vi "Autocycle v0.1.vi"(6 "start time":timestamp, 7 "Message Queue":refnum<queue>, 8 "error in":errorcluster, 9 "Run Time in":dbl, 10 "Auto Para":T1={"Agitator Delays"=[], "TF Delays"=[], "Insertion Delays"=[], "Cutting Delays"=[], "PF Delays"=[], "Measur. Delays"=[1000.0], "Reject Delays"=[1000], "BF Delays"=[1000]}, 11 "Counts in":cluster{"OutputCount":u32, "RejectCount":u32}) -> (0 "error out":errorcluster, 1 "Run Time out":dbl, 3 "Counts out":cluster{"OutputCount":u32, "RejectCount":u32})   [LabVIEW 2017]
uses:
  Controls/Auto Delays.ctl
  support/Message Queue/Message Cluster.ctl
  Controls/Auto Times.ctl
  Global Variables/RT GV.vi
  Global Variables/FPGA GV.vi
  <vilib>/Utility/error.llb/Error Cluster From Error Code.vi
  <vilib>/rvi/errors/niLvFpgaAdjustHostInterfaceError.vi
  support/Message Queue/Enqueue Message (Single).vi
  <vilib>/rvi/interface/nirviReadWriteControl/nirviReadWriteControl.xnode
  Controls/FPGA Ref.ctl
  NiFpgaLv.dll
  <vilib>/rvi/interface/Simulation/niFpgaSimulationCallBeginRW.vi
  support/Message Queue/Message Queue.lvlib
panel:
  in  "Max Successive":u32
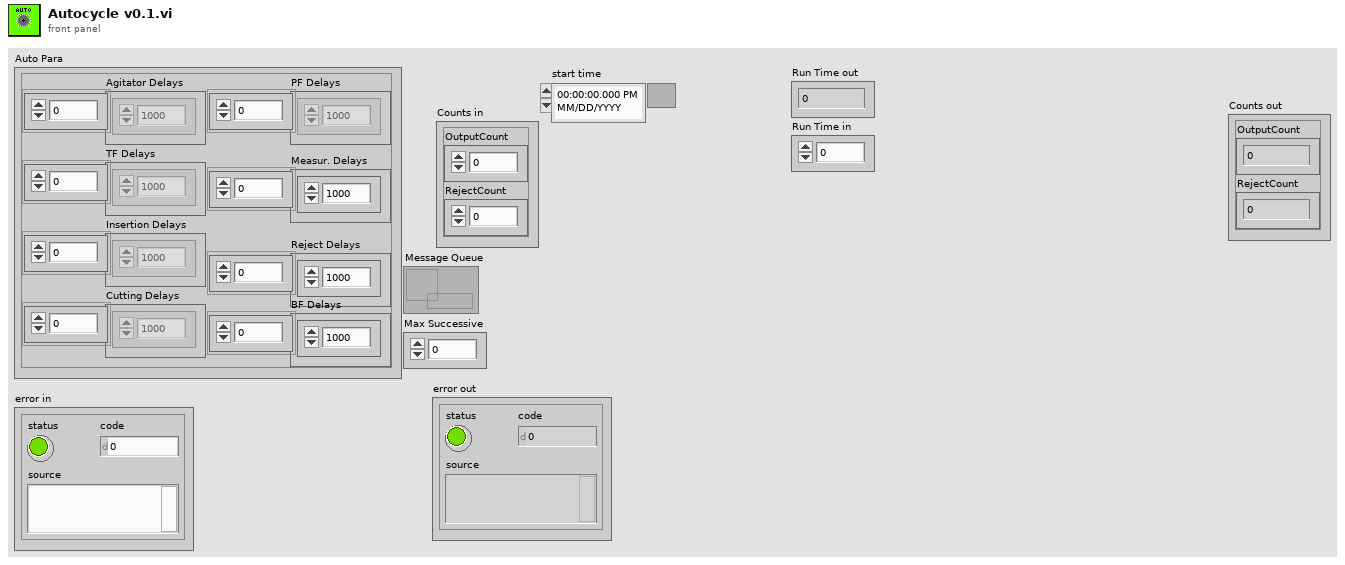
[diagram p1: front panel]
types:
  T1 = typedef "Auto Delays.ctl" = cluster{"Agitator Delays":u32[], "TF Delays":u32[], "Insertion Delays":u32[], "Cutting Delays":u32[], "PF Delays":u32[], "Measur. Delays":dbl[], "Reject Delays":u32[], "BF Delays":u32[]}
  T2 = cluster{"Tube Present":bool[], "Output Count":u32}
  T3 = typedef "FPGA Ref.ctl" = refnum<k20>
  T4 = cluster{"TL_Red":bool, "TL_Orange":bool, "TL_Green":bool, "TL_Buzzer":bool, "SOL_Index_Rotary_CW":bool, "SOL_Index_CNVR_Rotary_CCW":bool, "SOL_Index_CNVR_Stopper_Rear":bool, "SOL_Index_CNVR_Output _Separator _Rear":bool, "Bowl Feeder_ ON1":bool, "Pump_CNVR_Motor _ON":bool, "SOL_PC_Gating_CYL_Rear":bool, "SOL_Tube_Feed_Agitatator":bool, "SOL_Tube_Feed_Gating_CYL":bool, "SOL_Insertion _CYL":bool, "SOL_Insertion_Clamp_CYL":bool, "SOL_Cutting_CYL":bool, "SOL_Cutting_Clamp_CYL":bool, "SOL_Insertion_Air_Nozzle":bool, "SOL_Measurement_CYL":bool, "DO1.19":bool, "SOL_Rejection CYL_1":bool, "SOL_Rejection CYL_2":bool, "SOL_Rejection CYL_3":bool, "SOL_Rejection CYL_4":bool, "Bowl Feeder_ON2":bool, "SOL_BF_BlowerON":bool, "SOL_BF1_Track1":bool, "SOL_BF1_Track2":bool, "SOL_BF2_Track1":bool, "SOL_BF2_Track2":bool, "DO1.30":bool, "DO1.31":bool}
  T5 = cluster{"Indexes":i32, "seconds since 1Jan1904":timestamp}
  T6 = typedef "Auto Times.ctl" = cluster{"Index Time":u32, "TF Time":u32, "Insertion Time":u32, "Cutting Time":u32, "PF Time":u32, "Meas. Time":u32, "Reject Time":u32}
  T7 = cluster{"Reject 1":bool, "Reject 2":bool, "Reject 3":bool, "Reject 4":bool}
  T8 = cluster{"Tube Present":bool[], "Parts Count":u32}
  T9 = cluster{"seconds since 1Jan1904":timestamp, "Auto Times":T6, "start time":timestamp}
  T10 = cluster{"Reject Pallets":cluster{"Reject 1":bool, "Reject 2":bool, "Reject 3":bool, "Reject 4":bool}, "Measurements":cluster{"1":dbl, "2":dbl, "3":dbl, "4":dbl}}
  T11 = typedef "Auto Stats.ctl" = cluster{"Time":timestamp, "OEE":cluster{"AVL":dbl, "PRF":dbl, "QUA":dbl, "OEE":dbl}, "Auto Times":T6, "Counts out":cluster{"OutputCount":u32, "RejectCount":u32}, "Measurements":cluster{"1":dbl, "2":dbl, "3":dbl, "4":dbl}, "Outputs":cluster{"OutputCount":u32, "Numeric Control":u32}}
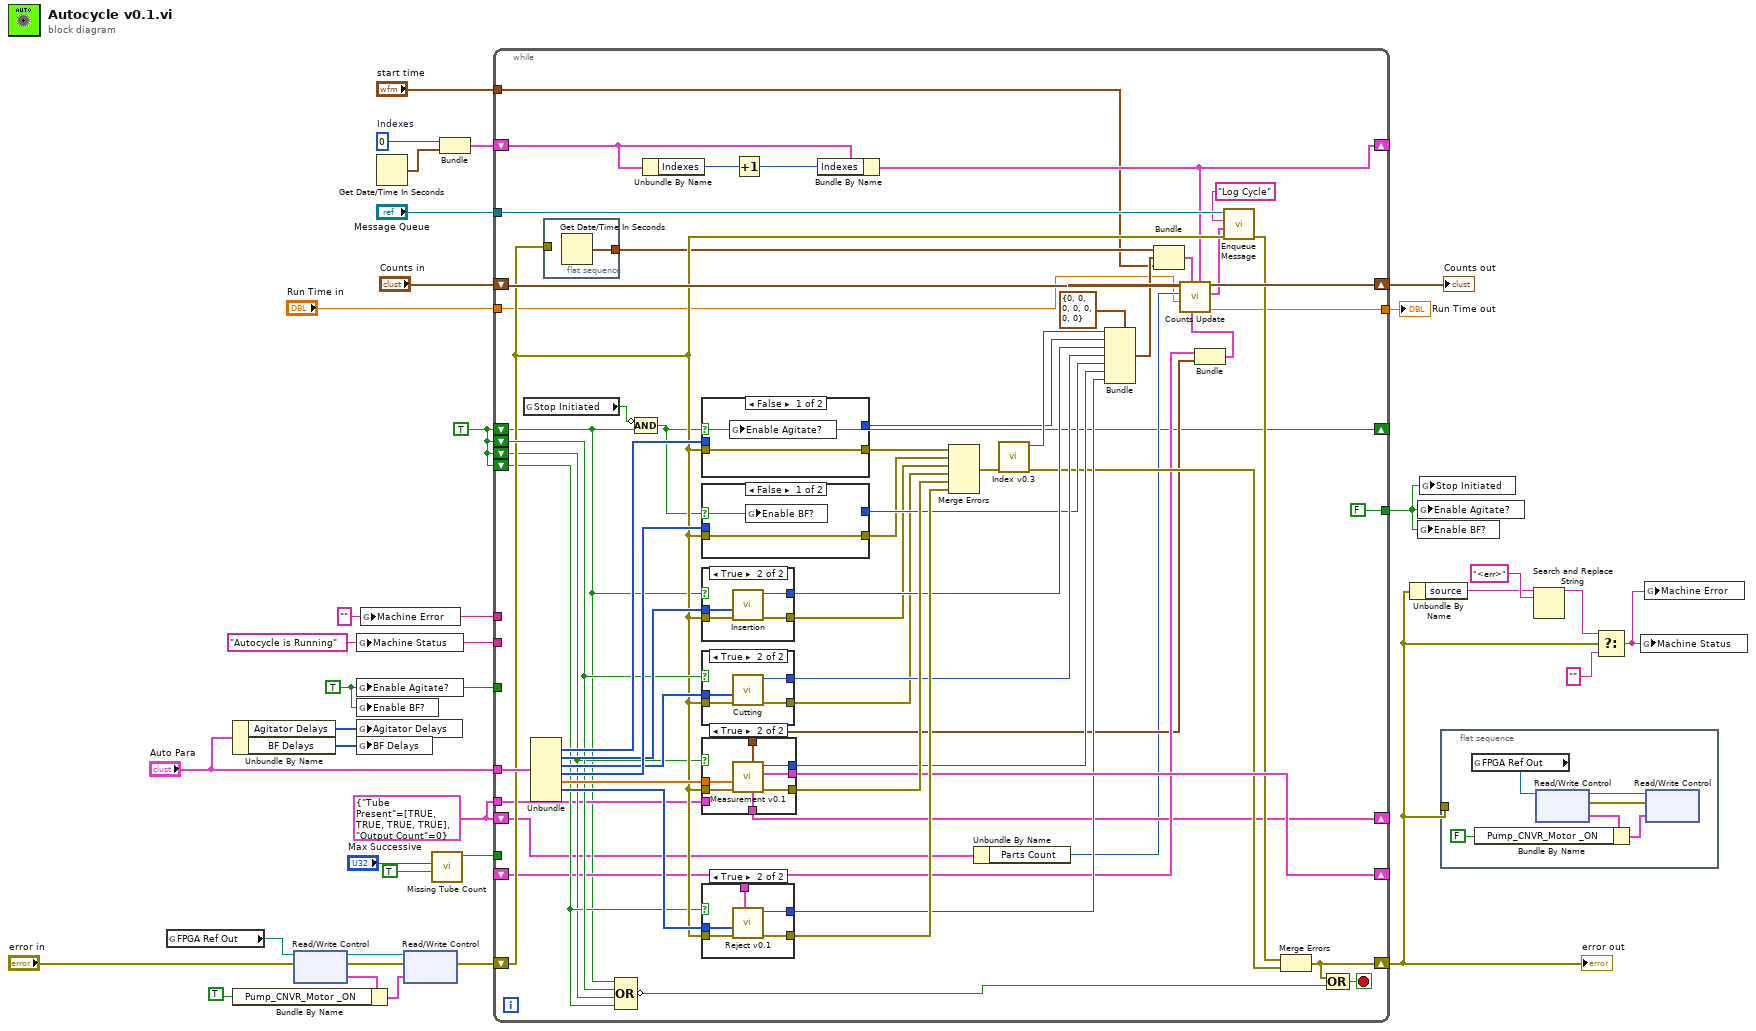
[diagram p0: block diagram]
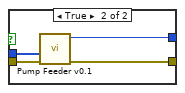
[diagram p2: hidden frame]
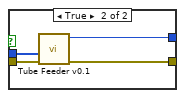
[diagram p5: hidden frame]
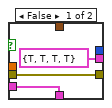
[diagram p7: hidden frame]
diagram:
  w7 = T2 {"Tube Present"=[TRUE, TRUE, TRUE, TRUE], "Output Count"=0} ("Part Count")
  w8 = "" ("Machine Error")
  w13 = 0  # Indexes
  w19 = "Autocycle is Running" ("Machine Status")
  w30 = TRUE ("Enable Agitate?")
  w20 = TRUE
  n1 = global read "FPGA GV.vi" "FPGA Ref Out"() -> (w29:T3)
  n2 = Unbundle By Name("Auto Para") -> ("Agitator Delays"=w32:u32[], "BF Delays"=w31:u32[])
  n3 = xnode "Read/Write Control"("FPGA VI Reference In"=w29, "error in"="error in") -> ("FPGA VI Reference Out"=w24:T3, "error out"=w25:errorcluster, "DO 1"=w28:T4)
  n4 = Bundle By Name(cluster=w28, "Pump_CNVR_Motor _ON"=TRUE) -> (w27:T4)
  n5 = global write "RT GV.vi" "Machine Status"(w19) -> ()
  n6 = global write "RT GV.vi" "Enable Agitate?"(w30) -> ()
  n7 = global write "RT GV.vi" "Enable BF?"(w30) -> ()
  n8 = global write "RT GV.vi" "Agitator Delays"(w32) -> ()
  n9 = global write "RT GV.vi" "BF Delays"(w31) -> ()
  n10 = global write "RT GV.vi" "Machine Error"(w8) -> ()
  n11 = Get Date/Time In Seconds() -> (seconds since 1Jan1904=w12:timestamp)
  n12 = xnode "Read/Write Control"("FPGA VI Reference In"=w24, "error in"=w25, "DO 1"=w27) -> ("error out"=w22:errorcluster)  [unwired: 1 out]
  n13 = call "Missing Tube Count.vi"("ResetMT?"=TRUE, "Max Successive"="Max Successive") -> ("Boolean"=w1:bool)  [unwired: 9 in]
  n14 = Bundle("Indexes"=w13, "seconds since 1Jan1904"=w12) -> (w11:T5)  [unwired: 1 in]
  n15 = while {
    tunnel: "Auto Para" -> [w89]
    shift-right: [w60] -> w17
    shift-left: w22 -> [w62]
    shift-right: [w83] -> _
    shift-left: _ -> [w54]
    shift-right: [w41] -> _
    shift-left: w20 -> [w40]
    shift-left: w20 -> [w63]
    shift-left: w20 -> [w56]
    shift-left: w20 -> [w57]
    shift-right: [w80] -> w35
    shift-left: "Counts in" -> [w79]
    tunnel: w30 -> [_]
    tunnel: "Message Queue" -> [w69]
    tunnel: [FALSE] -> w10
    tunnel: w19 -> [_]
    shift-right: [w45] -> _
    shift-left: w11 -> [w50]
    tunnel: w8 -> [_]
    shift-right: [w43] -> _
    shift-left: w7 -> [w39]
    tunnel: w7 -> [w44]
    tunnel: "start time" -> [w38]
    tunnel: [w37] -> w5
    tunnel: "Run Time in" -> [w36]
    tunnel: w1 -> [_]
    stop <- w81 stop-if-true
    n16 = global read "RT GV.vi" "Stop Initiated"() -> (w70:bool)
    n17 = Unbundle(w89) -> ("TF Delays"=w92:u32[], "Insertion Delays"=w91:u32[], "Cutting Delays"=w90:u32[], "PF Delays"=w93:u32[], "Measur. Delays"=w87:dbl[], "Reject Delays"=w85:u32[])  [unwired: 2 out]
    n18 = flat-sequence {
      tunnel: w62 -> [_]
      tunnel: [w94] -> w48
      frame #0 {
        n19 = Get Date/Time In Seconds() -> (seconds since 1Jan1904=w94:timestamp)
      }
    }
    n20 = Compound Arithmetic op=OR(w40, w63, w56, w57) -> (invert w82:bool)
    n21 = Compound Arithmetic op=AND(invert w70, w40) -> (w41:bool)
    n22 = Unbundle By Name(w50) -> ("Indexes"=w51:i32)
    n23 = case shown="False" w41 {
      selector: w41 -> [w111 _]
      tunnel: w62 -> [w112 w116]
      tunnel: [w112 w115] -> w88
      tunnel: w92 -> [_ w114]
      tunnel: [_ w113] -> w77
      frame False {
        n24 = global write "RT GV.vi" "Enable Agitate?"(w111) -> ()
      }
      frame True {
        n25 = call "Tube Feeder v0.1.vi"("error in (no error)"=w116, "TF Para"=w114) -> ("error out"=w115:errorcluster, "TF Time"=w113:u32)  [unwired: 8 in]
      }
    }
    n26 = case shown="False" w41 {
      selector: w41 -> [w95 _]
      tunnel: w62 -> [w96 w100]
      tunnel: [w96 w99] -> w65
      tunnel: w93 -> [_ w98]
      tunnel: [_ w97] -> w74
      frame False {
        n27 = global write "RT GV.vi" "Enable BF?"(w95) -> ()
      }
      frame True {
        n28 = call "Pump Feeder v0.1.vi"("error in (no error)"=w100, "TF Delays"=w98) -> ("error out"=w99:errorcluster, "PF Time"=w97:u32)  [unwired: 8 in]
      }
    }
    n29 = case shown="True" w40 {
      tunnel: w62 -> [w106 w110]
      tunnel: [w106 w109] -> w66
      tunnel: w91 -> [_ w108]
      tunnel: [_ w107] -> w76
      frame False {
      }
      frame True {
        n30 = call "Insertion.vi"("error in (no error)"=w110, "Insertion Delays"=w108) -> ("error out"=w109:errorcluster, "Insertion Time"=w107:u32)  [unwired: 7 in, 1 out]
      }
    }
    n31 = case shown="True" w63 {
      tunnel: w62 -> [w101 w105]
      tunnel: [w101 w104] -> w67
      tunnel: w90 -> [_ w103]
      tunnel: [_ w102] -> w75
      frame False {
      }
      frame True {
        n32 = call "Cutting.vi"("error in (no error)"=w105, "Cutting Delays"=w103) -> ("error out"=w104:errorcluster, "Cutting Time"=w102:u32)  [unwired: 8 in]
      }
    }
    n33 = case shown="True" w56 {
      tunnel: w62 -> [w125 w132]
      tunnel: [w125 w131] -> w86
      tunnel: w87 -> [_ w130]
      tunnel: [_ w129] -> w73
      tunnel: [_ w128] -> w53
      tunnel: [T7 {"Reject 1"=TRUE, "Reject 2"=TRUE, "Reject 3"=TRUE, "Reject 4"=TRUE} ("Reject Pallets") w127] -> w83
      tunnel: [w123 w126] -> w43
      tunnel: w44 -> [w123 _]
      frame False {
      }
      frame True {
        n34 = call "Measurement v0.1.vi"("error in (no error)"=w132, "TF Delays"=w130) -> ("error out"=w131:errorcluster, "Reject Pallets"=w127:T7, "PF Time"=w129:u32, "Part Count"=w126:T8, "Measurements"=w128:cluster{"1":dbl, "2":dbl, "3":dbl, "4":dbl})  [unwired: 5 in]
      }
    }
    n35 = case shown="True" w57 {
      tunnel: w62 -> [w117 w122]
      tunnel: [w117 w121] -> w84
      tunnel: w85 -> [_ w120]
      tunnel: [_ w119] -> w72
      tunnel: w54 -> [_ w118]
      frame False {
      }
      frame True {
        n36 = call "Reject v0.1.vi"("Reject Pallets"=w118, "error in (no error)"=w122, "TF Delays"=w120) -> ("error out"=w121:errorcluster, "PF Time"=w119:u32)  [unwired: 7 in]
      }
    }
    n37 = Increment(x=w51) -> (x+1=w49:i32)
    n38 = Bundle By Name(cluster=w50, "Indexes"=w49) -> (w45:T5)
    n39 = Merge Errors(w88, w65, w66, w67, w86, w84) -> (w61:errorcluster)
    n40 = Unbundle By Name(w39) -> ("Parts Count"=w42:u32)
    n41 = call "Index v0.3.vi"("error in (no error)"=w61) -> ("error out"=w59:errorcluster, "Index Time"=w78:u32)  [unwired: 7 in, 2 out]
    n42 = Bundle(cluster=T6 {"Index Time"=0, "TF Time"=0, "Insertion Time"=0, "Cutting Time"=0, "PF Time"=0, "Meas. Time"=0, "Reject Time"=0} ("Auto Times"), "Index Time"=w78, "TF Time"=w77, "Insertion Time"=w76, "Cutting Time"=w75, "PF Time"=w74, "Meas. Time"=w73, "Reject Time"=w72) -> (w47:T6)
    n43 = Bundle("seconds since 1Jan1904"=w48, "Auto Times"=w47, "start time"=w38) -> (w46:T9)  [unwired: 1 in]
    n44 = Bundle("Reject Pallets"=w54, "Measurements"=w53) -> (w52:T10)  [unwired: 1 in]
    n45 = call "Counts Update.vi"("Perf"=w45, "output cluster"=w52, "Cluster"=w46, "Previous Run Time"=w36, "Parts Count"=w42, "Counts in"=w79) -> ("Run Time"=w37:dbl, "Auto Stats"=w55:T11, "Counts out"=w80:cluster{"OutputCount":u32, "RejectCount":u32})  [unwired: 2 in, 1 out]
    n46 = call-poly "Enqueue Message.vi"("error in (no error)"=w62, "Message Data"=w55, "Message"="Log Cycle", "Message Queue"=w69) -> ("error out"=w58:errorcluster)  [unwired: 6 in, 1 out]
    n47 = Merge Errors(w58, w59) -> (w60:errorcluster)
    n48 = Compound Arithmetic op=OR(w60, w82) -> (w81:bool)
  }
  "error out" <- w17
  "Counts out" <- w35
  "Run Time out" <- w5
  n49 = Unbundle By Name(w17) -> ("source"=w15:string)
  n50 = global write "RT GV.vi" "Enable Agitate?"(w10) -> ()
  n51 = global write "RT GV.vi" "Enable BF?"(w10) -> ()
  n52 = global write "RT GV.vi" "Stop Initiated"(w10) -> ()
  n53 = flat-sequence {
    tunnel: w17 -> [_]
    frame #0 {
      n54 = global read "FPGA GV.vi" "FPGA Ref Out"() -> (w133:T3)
      n55 = xnode "Read/Write Control"("FPGA VI Reference In"=w133) -> ("FPGA VI Reference Out"=w138:T3, "error out"=w137:errorcluster, "DO 1"=w135:T4)  [unwired: 1 in]
      n56 = Bundle By Name(cluster=w135, "Pump_CNVR_Motor _ON"=FALSE) -> (w136:T4)
      n57 = xnode "Read/Write Control"("FPGA VI Reference In"=w138, "error in"=w137, "DO 1"=w136) -> ()  [unwired: 2 out]
    }
  }
  n58 = Search and Replace String(input string=w15, search string="<err>") -> (result string=w14:string)  [unwired: 6 in, 3 out]
  n59 = Select(t=w14, s=w17, f="" ("Machine Status")) -> (s? t:f=w9:string)
  n60 = global write "RT GV.vi" "Machine Status"(w9) -> ()
  n61 = global write "RT GV.vi" "Machine Error"(w9) -> ()
